vi "Drive Published Globals.vi"() -> ()   [LabVIEW 2015]
panel:
  out "Drive Finished Operation":bool
  # "Tip: The global is a good way publish state or\ninformational/debugging values.\nIt is not  advised that you put setpoint values here."
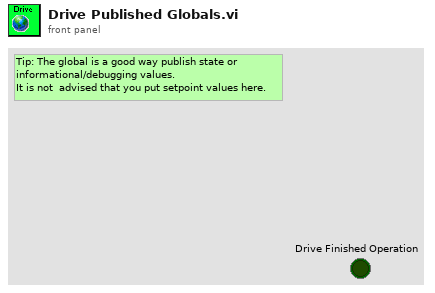
[diagram p1: front panel]
diagram:
